vi "Auto_Conf.vi"() -> ()   [LabVIEW 2015]
panel:
  in  "Has Turned":bool
  in  "AutoToRun":u8
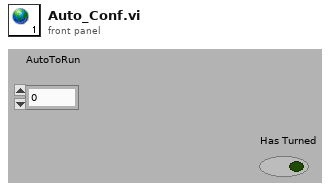
[diagram p1: front panel]
diagram:
